vi "TC-handler.vi"(10 "read buffer in":string) -> (3 "Thermocouple Inputs (degC)":T1)   [LabVIEW 2020]
uses:
  <vilib>/regexp/Match Regular Expression.xnode
  controls/thermocouple-input-cluster.ctl
panel:
  out "x <= y?":bool
  out "offset past match":i32
  out "concatenated string":string
  out "match + rest of string":string
  in  "search string/char (-)":string="[+-]"
  out "prototype array":dbl[](array[numeric])
  out "too big cluster":T2
  out "data array":dbl[](array[numeric])
  in  "delimiter (Tab)":string=","
  in  "format string":string
  out "substring":string
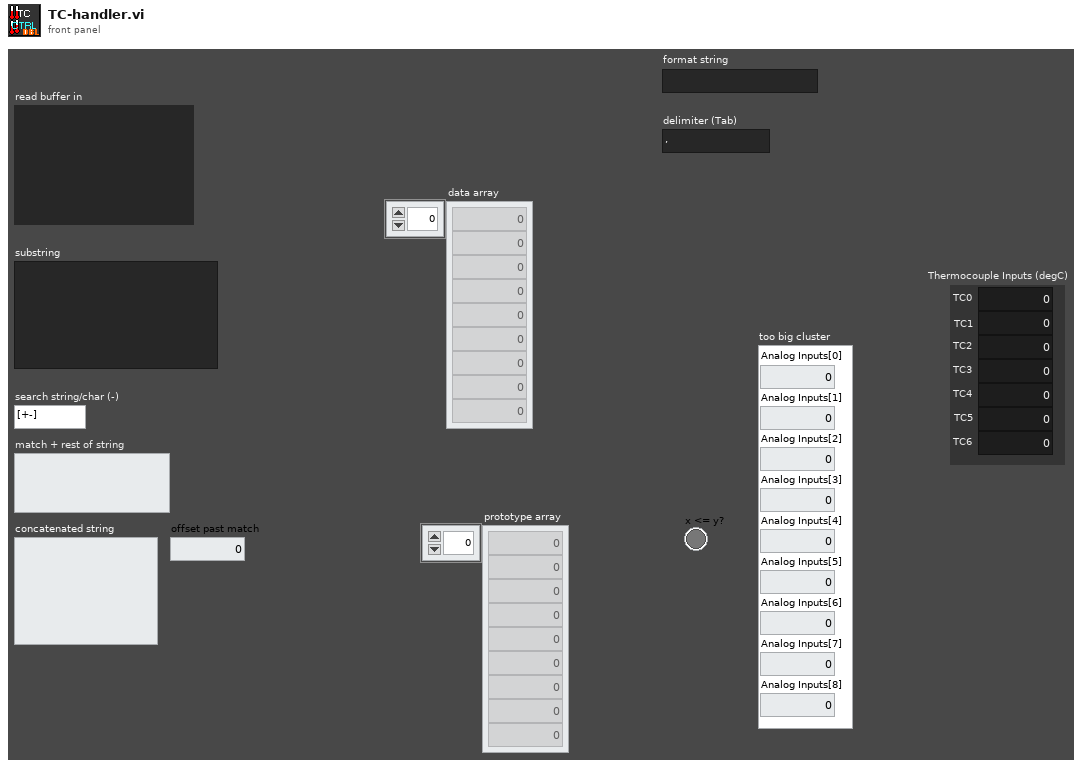
[diagram p1: front panel]
types:
  T1 = typedef "thermocouple-input-cluster.ctl" = cluster{"TC0":dbl, "TC1":dbl, "TC2":dbl, "TC3":dbl, "TC4":dbl, "TC5":dbl, "TC6":dbl}
  T2 = cluster{"Analog Inputs[0]":dbl, "Analog Inputs[1]":dbl, "Analog Inputs[2]":dbl, "Analog Inputs[3]":dbl, "Analog Inputs[4]":dbl, "Analog Inputs[5]":dbl, "Analog Inputs[6]":dbl, "Analog Inputs[7]":dbl, "Analog Inputs[8]":dbl}
  T3 = cluster{"Thermocouple Inputs (degC)[0]":dbl, "Thermocouple Inputs (degC)[1]":dbl, "Thermocouple Inputs (degC)[2]":dbl, "Thermocouple Inputs (degC)[3]":dbl, "Thermocouple Inputs (degC)[4]":dbl, "Thermocouple Inputs (degC)[5]":dbl, "Thermocouple Inputs (degC)[6]":dbl, "Thermocouple Inputs (degC)[7]":dbl, "Thermocouple Inputs (degC)[8]":dbl}
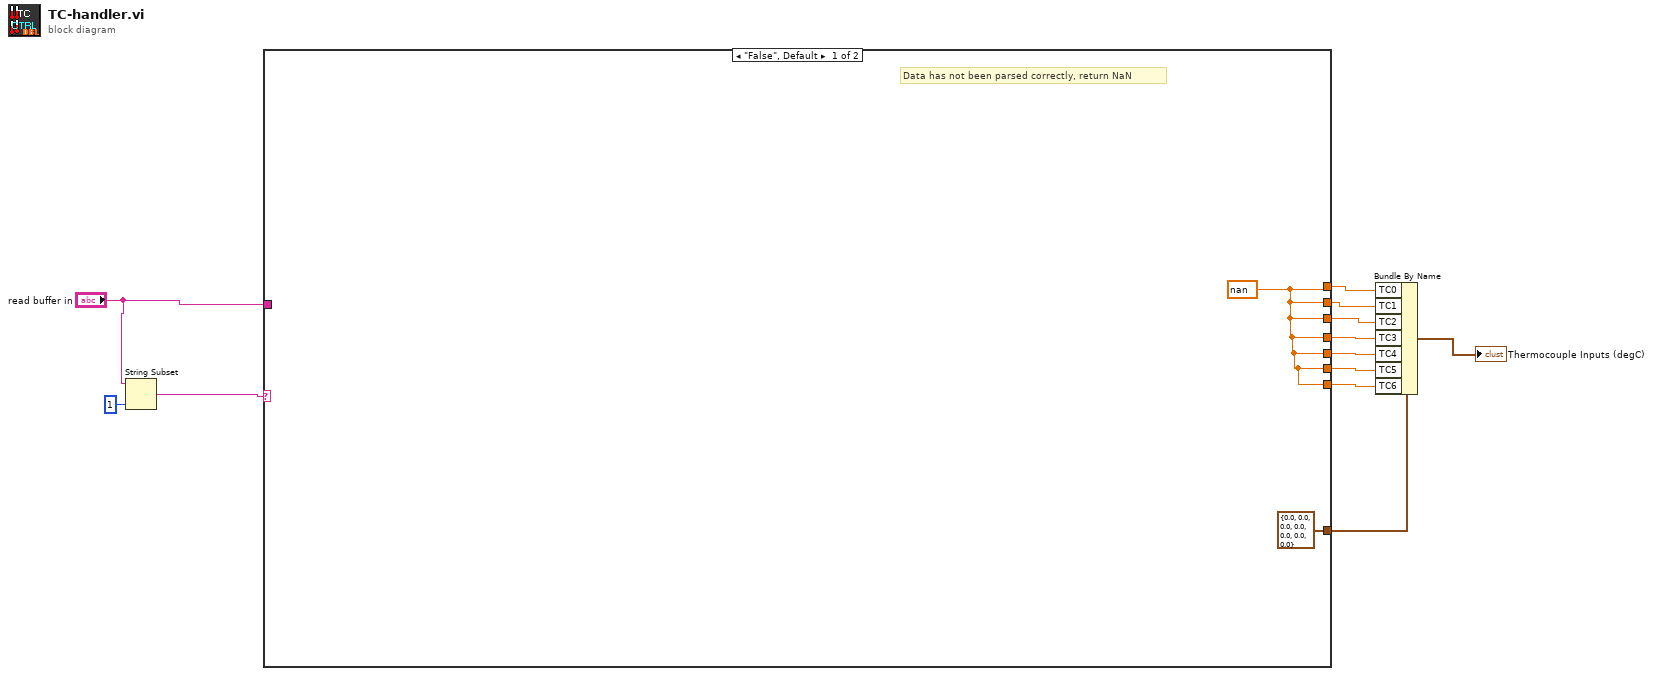
[diagram p0: block diagram]
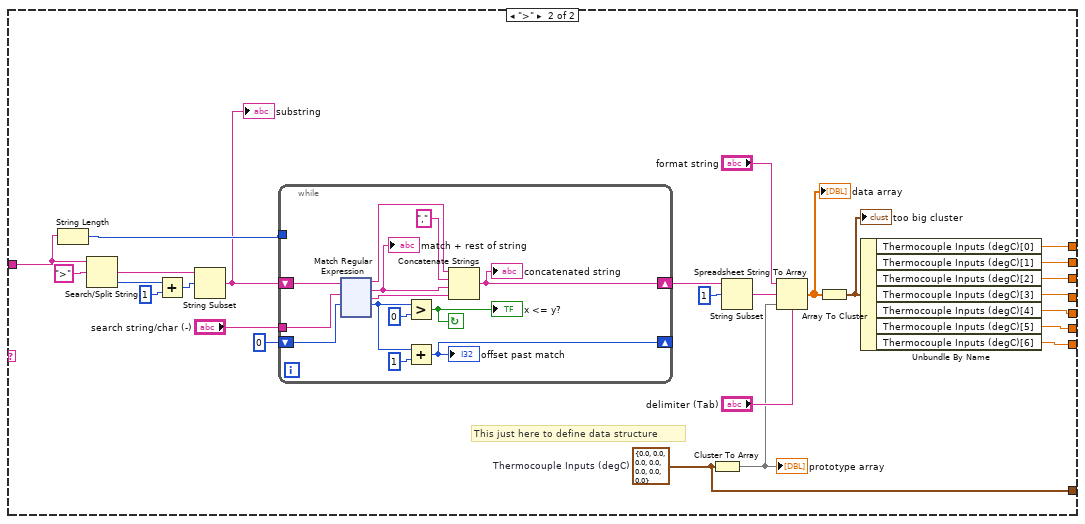
[diagram p2: hidden frame]
diagram:
  n1 = String Subset(string="read buffer in", length (rest)=1 ("length (rest)")) -> (substring=w1:string)  [unwired: 1 in]
  n2 = case shown="\"False\", Default" w1 {
    tunnel: "read buffer in" -> [_ w31]
    tunnel: [w14 w25] -> w12
    tunnel: [w14 w24] -> w11
    tunnel: [w14 w23] -> w10
    tunnel: [w14 w22] -> w9
    tunnel: [w14 w21] -> w8
    tunnel: [w14 w20] -> w7
    tunnel: [w14 w19] -> w6
    tunnel: [T1 {"TC0"=0.0, "TC1"=0.0, "TC2"=0.0, "TC3"=0.0, "TC4"=0.0, "TC5"=0.0, "TC6"=0.0} ("Thermocouple Inputs (degC)") w15] -> w5
    frame "False", Default {
      w14 = nan
      # "Data has not been parsed correctly, return NaN"
    }
    frame ">" {
      w15 = T1 {"TC0"=0.0, "TC1"=0.0, "TC2"=0.0, "TC3"=0.0, "TC4"=0.0, "TC5"=0.0, "TC6"=0.0}  # Thermocouple Inputs (degC)
      # "This just here to define data structure"
      n3 = String Length(string=w31) -> (length=w30:i32)
      n4 = Search/Split String(string=w31, search string/char (-)=">") -> (match + rest of string=w35:string, offset of match=w36:i32)  [unwired: 1 in, 1 out]
      n5 = Add(x=w36, y=1) -> (x+y=w38:i32)
      n6 = String Subset(string=w35, offset (0)=w38) -> (substring=w27:string)  [unwired: 1 in]
      "substring" <- w27
      n7 = while {
        tunnel: w30 -> [_]
        tunnel: "search string/char (-)" -> [w53]
        shift-right: [w45] -> _
        shift-left: 0 ("offset past match") -> [w48]
        shift-right: [w50] -> w17
        shift-left: w27 -> [w47]
        stop <- w42 continue-if-true
        n8 = xnode ("Match Regular Expression")("input string"=w47, "regular expression"=w53, "offset (0)"=w48) -> ("before match"=w41:string, "whole match"=w52:string, "after match"=w51:string, "offset past match"=w43:i32)  [unwired: 3 in, 1 out]
        "match + rest of string" <- w52
        n9 = Greater?(x=w43, y=0) -> (0:w42:bool)
        "x <= y?" <- w42
        n10 = Add(x=w43, y=1) -> (x+y=w45:i32)
        "offset past match" <- w45
        n11 = Concatenate Strings(w41, "," ("string"), w52, w51) -> (w50:string)
        "concatenated string" <- w50
      }
      n12 = Cluster To Array(cluster=w15) -> (array=w33:dbl[])
      "prototype array" <- w33
      n13 = String Subset(string=w17, offset (0)=1) -> (substring=w16:string)  [unwired: 1 in]
      n14 = Spreadsheet String To Array(delimiter (Tab)="delimiter (Tab)", format string="format string", spreadsheet string=w16, array type (2D Dbl)=w33) -> (array=w32:dbl[])
      "data array" <- w32
      n15 = Array To Cluster(array=w32) -> (cluster=w26:T3)
      "too big cluster" <- w26
      n16 = Unbundle By Name(w26) -> ("Thermocouple Inputs (degC)[0]"=w25:dbl, "Thermocouple Inputs (degC)[1]"=w24:dbl, "Thermocouple Inputs (degC)[2]"=w23:dbl, "Thermocouple Inputs (degC)[3]"=w22:dbl, "Thermocouple Inputs (degC)[4]"=w21:dbl, "Thermocouple Inputs (degC)[5]"=w20:dbl, "Thermocouple Inputs (degC)[6]"=w19:dbl)
    }
  }
  n17 = Bundle By Name(cluster=w5, "TC0"=w12, "TC1"=w11, "TC2"=w10, "TC3"=w9, "TC4"=w8, "TC5"=w7, "TC6"=w6) -> (→"Thermocouple Inputs (degC)":T1)
